vi "UHR-Fleezers Control (host) - 10.8.vi"() -> ()   [LabVIEW 2014] (continued)
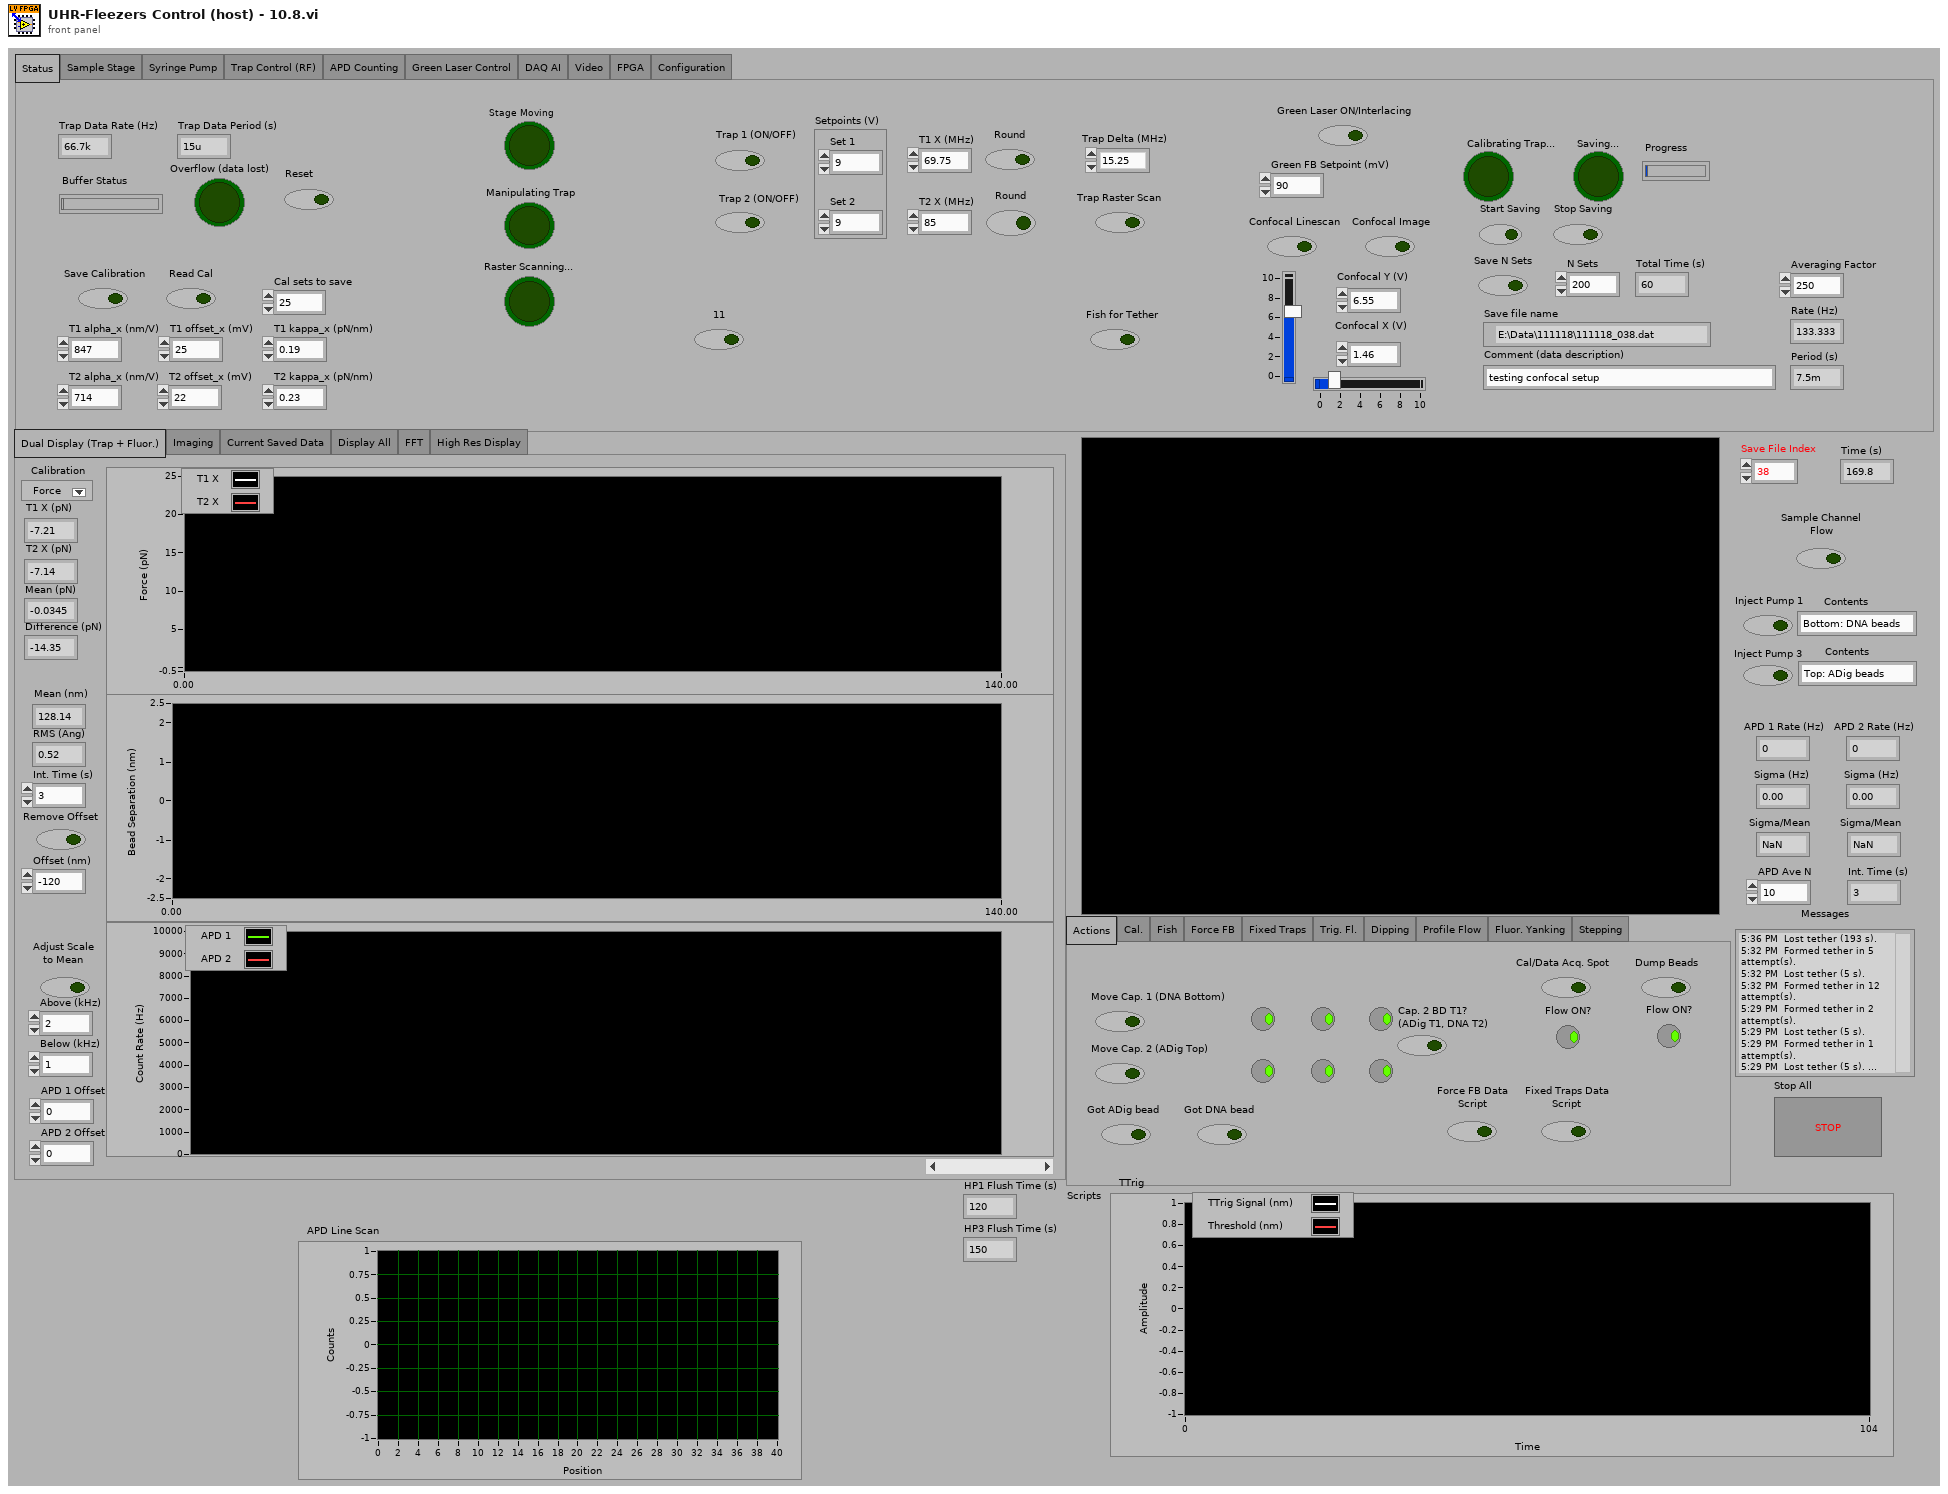
[diagram p1: front panel]
types:
  T1 = enum32{"Actions", "Cal.", "Fish", "Force FB", "Fixed Traps", "Trig. Fl.", "Dipping", "Profile Flow", "Fluor. Yanking", "Stepping"}
  T2 = typedef "IMAQ Image.ctl" = refnum<image>
  T3 = enum32{"Dual Display (Trap + Fluor.)", "Imaging", "Current Saved Data", "Display All", "FFT", "High Res Display"}
  T4 = enum32{"Status", "Sample Stage", "Syringe Pump", "Trap Control (RF)", "APD Counting", "Green Laser Control", "DAQ AI", "Video", "FPGA", "Configuration"}
  T5 = cluster{"Pump 1":cluster{"Diameter (mm)":dbl, "Units":dbl, "Volume":dbl, "Rate":dbl}, "Pump 2":cluster{"Diameter (mm)":dbl, "Units":dbl, "Volume":dbl, "Rate":dbl}, "Pump 3":cluster{"Diameter (mm)":dbl, "Units":dbl, "Volume":dbl, "Rate":dbl}}
  T6 = enum32{"IR Laser Interlacing (Direct RF Board Control Method)", "AOD Raster Scan", "Feedback on Trap Intensity", "Feedback on Trap Position"}
  T7 = typedef "LVPoint32TypeDef.ctl" = cluster{"Horizontal":i32, "Vertical":i32}
  T8 = cluster{"Scan Range AOD (nm) 2":dbl, "Step Size AOD (nm) 2":dbl, "Scan Speed AOD (nm/s) 2":dbl, "Number of scans (AOD) 2":u16, "Label":string}[]
  T9 = cluster{"Set 1":cluster{"proportional gain (Kc)":i16, "integral gain (Kc*Ts/Ti)":i16, "derivative gain (Kc*Td/Ts)":i16}, "Set 2":cluster{"proportional gain (Kc)":i16, "integral gain (Kc*Ts/Ti)":i16, "derivative gain (Kc*Td/Ts)":i16}}
  T10 = cluster{"Trap 1":fxp<+/-,16,1>, "Trap 2":fxp<+/-,16,1>}
  T11 = cluster{"proportional gain (Kc)":fxp<+/-,16,8>, "integral gain (Kc*Ts/Ti)":fxp<+/-,16,8>, "derivative gain (Kc*Td/Ts)":fxp<+/-,16,8>}
  T12 = cluster{"output high":fxp<+/-,16,1>, "output low":fxp<+/-,16,1>}
  T13 = cluster{"Set 1":fxp<+/-,16,1>, "Set 2":fxp<+/-,16,1>}
  T14 = cluster{"proportional gain (Kc)":i16, "integral gain (Kc*Ts/Ti)":i16, "derivative gain (Kc*Td/Ts)":i16}
  T15 = cluster{"Set 1":bool, "Set 2":bool, "Set 3":bool}
  T16 = typedef "LVMinMaxIncTypeDef.ctl" = cluster{"Minimum":dbl, "Maximum":dbl, "Increment":dbl}
  T17 = typedef "Image Type" = u32
  T18 = typedef "nirio_resource_hc.ctl" = tag
  T19 = typedef "openfpgaref.8.6.ctl" = refnum<k20>
  T20 = cluster{"New Image":T2, "New Image":T2, "New Image":T2, "New Image":T2}
  T21 = typedef "XDNodeRunTimeDep.lvlib/timing_clust.ctl" = cluster{"Expected End [f-1]":u64, "Actual End [f-1]":u64, "Finished Late? [f-1]":bool, "Expected End [i-1]":u64, "Actual End [i-1]":u64, "Finished Late? [i-1]":bool, "Expected Start [i]":u64, "Actual Start [i]":u64, "Expected Start [f]":u64, "Actual Start [f]":u64, "Source Name":string, "Structure Name":string, "Period":i64, "Deadline":i64, "Offset":i64, "Start":i64, "Priority":i32, "Timeout":i32, "Mode":T22, "Wakeup Reason":T23, "Error":errorcluster, "Source Type":string, "Secondary Source Type":string, "Global End Time":u64, "Global Start Time":u64, "Frame Duration":u64, "Iteration Duration":u64, "Assigned CPU":i32, "I/O Scan Engine Mode":u32}
  T22 = typedef "XDNodeRunTimeDep.lvlib/nitl_modes.ctl" = enum32{"No Change", "Process missed periods, maintain original phase", "Discard missed periods, maintain original phase", "Process missed periods, ignore original phase", "Discard missed periods, ignore original phase"}
  T23 = typedef "XDNodeRunTimeDep.lvlib/wakeup.ctl" = enum32{"Normal", "Aborted", "Asynchronous wakeup", "Timing source error", "Timed loop error", "Timeout"}
  T24 = enum16{"big-endian, network order", "native, host order", "little-endian"}
  T25 = enum16{"open", "replace", "create", "open or create", "replace or create", "replace or create with confirmation"}
  T26 = cluster{"Scan Range AOD (nm) 2":dbl, "Step Size AOD (nm) 2":dbl, "Scan Speed AOD (nm/s) 2":dbl, "Number of scans (AOD) 2":u16, "Label":string}
  T27 = cluster{"[0]":dbl, "[1]":dbl, "[2]":dbl, "[3]":dbl, "[4]":dbl, "[5]":dbl}
  T28 = cluster{"Diameter (mm)":dbl, "Units":dbl, "Volume":dbl, "Rate":dbl}
  T29 = cluster{"Left":i32, "Top":i32, "Width":u32, "Height":u32}
  T30 = cluster{cluster{"Left":i32, "Top":i32, "Width":u32, "Height":u32}}[]
  T31 = enum32{"setting", "request", "request control", "info", "statistics", "system settings", "I/O sub system", "HRT control", "camera descriptions", "device specific data", "event sub system settings", "event sub system results", "image memory manager"}
  T32 = typedef "AviRefnum.ctl" = refnum<k1>
  T33 = typedef "imagedata.ctl" = cluster{"image type":i32, "image depth":i32, "image":u8[], "mask":u8[], "colors":u32[], "Rectangle":cluster{"left":i16, "top":i16, "right":i16, "bottom":i16}}
  T34 = enum32{"Normal Display", "Dual Display (APD)", "FFT", "High Res Display"}
  T35 = cluster{"Origin Pixel":cluster{"X":sgl, "Y":sgl}, "Angle Relative to Horizontal (deg)":sgl, "Axis Reference":u32}
  T36 = typedef "Simple Grid Descriptor" = cluster{"X Step":sgl, "Y Step":sgl, "Unit":T37}
  T37 = typedef "Image Unit" = enum32{"Undefined", "Angström", "Micrometer", "Millimeter", "Centimeter", "Meter", "Kilometer", "Microinch", "Inch", "Feet", "Nautical miles", "Standard miles", "Steps"}
  T38 = cluster{"averaging mode":u16, "weighting mode":u16, "number of averages":u32}
  T39 = cluster{"dB On (F)":bool, "unwrap phase (F)":bool, "convert to degree (F)":bool}
  T40 = cluster{string, string, string, string, string, string, string, string}
  T41 = cluster{string, string, string, string, string, string, string, string, string, string, string, string}
  T42 = cluster{string, string, string, string, string, string, string, string, string, string, string, string, string}
  T43 = cluster{string, string, string, string, string, string, string, string, string, string, string, string, string, string}
  T44 = cluster{"BD 1 Frequency 1 (MHz)":dbl, "BD 1 Frequency 2 (MHz)":dbl}
  T45 = cluster{"f0":dbl, "df":dbl, "magnitude":dbl[]}[][]
diagram:
  w6 = u16 20 items=["1.0"=10, "1.5"=15, "2.0"=20] ("stop bits (10: 1 bit)")
  w9 = u16 20 items=["1.0"=10, "1.5"=15, "2.0"=20] ("stop bits (10: 1 bit)")
  w67 = u16 20 items=["1.0"=10, "1.5"=15, "2.0"=20] ("stop bits (10: 1 bit)")
  w74 = T17 2 items=["Grayscale (U8)", "Grayscale (I16)", "Grayscale (SGL)", "Complex (CSG)", "RGB (U32)", "HSL (U32)", "RGB (U64)", "Grayscale (U16)"] ("Image Type")
  w137 = cluster{"output high":i16, "output low":i16} {"output high"=3000, "output low"=0} ("FB output range 1")
  w208 = 10.0 ("y")
  w207 = 32767.0 ("y")
  w223 = 6.0  # clock mult.
  w224 = 49152000.0  # TCXO frequ.
  # "Bottom 1 Harvard"
  # "Top 3 Harvard"
  # "Center Harvard"
  # "Bottom 1 Harvard"
  # "Top 3 Harvard"
  # "Center Harvard"
  n1 = Build Array("DIO count 1 (ticks)", "DIO count 2 (ticks)", "DIO count 3 (ticks)") -> (w124:u32[])
  n2 = local read "AO1"() -> (w202:dbl)
  n3 = local read "AO2"() -> (w201:dbl)
  n4 = local read "Scan Increment (MHz)"() -> (w219:dbl)
  n5 = local read "Continuous MCL Scanning"() -> (w189:bool)
  n6 = local read "Fast Scan Dir"() -> (w188:bool)
  n7 = local read "Number of scans (MCL)"() -> (w190:u64)
  n8 = property on="AI Count (ticks)" class="DigNum (strict)"("Val(Sgnl)"="AI Count (ticks)") -> ()  [unwired: 2 in, 2 out]
  n9 = Multiply(x=w202, y=w207) -> (x*y=w204:dbl)
  n10 = Multiply(x=w201, y=w207) -> (x*y=w206:dbl)
  n11 = Divide(x=w204, y=w208) -> (x/y=w203:dbl)
  n12 = Divide(x=w206, y=w208) -> (x/y=w205:dbl)
  n13 = To Word Integer(number=w203) -> (16bit integer=w200:i16)
  n14 = To Word Integer(number=w205) -> (16bit integer=w199:i16)
  n15 = Not(x=w188) -> (.not. x?=w183:bool)
  n16 = local read "Cycles/step (MCL)"() -> (w191:u64)
  n17 = Multiply(x=w219, y=1000.0) -> (x*y=w226:dbl)
  n18 = local read "Scan steps (MCL)"() -> (w192:u64)
  n19 = local write "Trap Pos FIFO Timeout"(u16 0 ("Trap Pos FIFO Timeout")) -> ()
  n20 = local read "Desired Scan Incr (V)"() -> (w194:dbl)
  n21 = Scale By Power Of 2(n=48, x=w226) -> (x*2^n=w227:dbl)
  n22 = Multiply(x=w224, y=w223) -> (x*y=w222:dbl)
  n23 = Divide(x=w227, y=w222) -> (x/y=w221:dbl)
  n24 = local read "Setpoints (V)"() -> (w240:cluster{"Set 1":dbl, "Set 2":dbl})
  n25 = To Quad Integer(1:w221) -> (0:w218:i64)
  n26 = Divide(x=40000000.0, y="AI Count (ticks)") -> (x/y=w179:dbl)
  n27 = Multiply(x=w194, y=32767.0) -> (x*y=w196:dbl)
  n28 = local read "Number Interlace Sets"() -> (w117:u8)
  n29 = Split 1D Array(array=w124, index=w117) -> (first subarray=w126:u32[])  [unwired: 1 out]
  n30 = Add Array Elements(numeric array=w126) -> (sum=w125:u32)
  n31 = local read "# Samples/channel"() -> (w211:u32)
  n32 = local read "Number of F/B Scans (AOD)"() -> (w212:u16)
  n33 = local read "Not-Interlacing Set"() -> (w116:enum32{"Set 1", "Set 2", "Set 3"})
  n34 = To Unsigned Byte Integer(number=w116) -> (unsigned 8bit integer=w122:u8)
  n35 = Index Array(array=w124, index=w122) -> (element=w123:u32)
  n36 = local read "Feedback On/Off"() -> (w243:cluster{"Set 1":bool, "Set 2":bool})
  n37 = local read "PID Gains"() -> (w235:T9)
  n38 = local read "Scan steps (AOD)"() -> (w217:u64)
  n39 = local read "All FB On/Off"() -> (w244:bool)
  n40 = local read "Cycles/step (AOD)"() -> (w216:u64)
  n41 = local write "AI rate (Hz)"(w179) -> ()
  n42 = Divide(x=w196, y=10.0) -> (x/y=w195:dbl)
  n43 = Multiply(x=w217, y=w216) -> (x*y=w215:u64)
  n44 = Multiply(x=3276.7, y=w240) -> (x*y=w239:cluster{"Set 1":dbl, "Set 2":dbl})
  n45 = xnode "FPGA Open VI Reference"("resource name"=T18 "750kHzDAQ") -> ("FPGA VI Reference Out"=w232:T19, "error out"=w231:errorcluster)  [unwired: 1 in]
  n46 = To Word Integer(number=w195) -> (16bit integer=w193:i16)
  n47 = Multiply(x=w215, y=u64 2) -> (x*y=w213:u64)
  n48 = local read "Sets to FIFO (Traps)"() -> (w247:T15)
  n49 = Divide(x=w179, y="FPGA Ave.") -> (x/y=w180:dbl)
  n50 = To Word Integer(number=w239) -> (16bit integer=w238:cluster{"Set 1":i16, "Set 2":i16})
  n51 = Unbundle By Name(w235) -> ("Set 1"=w234:T14, "Set 2"=w233:T14)
  n52 = Multiply(x=w213, y=w212) -> (x*y=w210:u64)
  n53 = local write "Ave. Rate (Hz)"(w180) -> ()
  n54 = Divide(x=w210, y=w211) -> (x/y=w209:dbl)
  n55 = Unbundle By Name(w238) -> ("Set 1"=w237:i16, "Set 2"=w236:i16)
  n56 = local read "2D or 1D Scan"() -> (w138:bool)
  n57 = local write "Data points/scans"(w210) -> ()
  n58 = local read "Scan BD"() -> (w228:bool)
  n59 = And(x=w243, y=w244) -> (x .and. y?=w242:cluster{"Set 1":bool, "Set 2":bool})
  n60 = local write "Data points/scan (f/b)"(w213) -> ()
  n61 = Reciprocal(x=w180) -> (1/x=w181:dbl)
  n62 = local read "N Acq Sets (Traps + Fl.)"() -> (w172:i16)
  n63 = local write "N sets should be saved"(w209) -> ()
  n64 = xnode "Invoke Method"("FPGA VI Reference In"=w232, "error in"=w231) -> ("FPGA VI Reference Out"=w136:T19, "error out"=w146:errorcluster)
  n65 = Unbundle By Name(w242) -> ("Set 1"=w246:bool, "Set 2"=w245:bool)
  n66 = local read "Interlace"() -> (w118:bool)
  n67 = Select(t=w125, s=w118, f=w123) -> (s? t:f=w115:u32)
  n68 = local write "Update Count (MCL)"(w115) -> ()
  n69 = local write "Total Counts (ticks)"(w115) -> ()
  n70 = local write "Ave. Period (s)"(w181) -> ()
  n71 = property on="2D or 1D Scan" class="Bool (strict)"("Val(Sgnl)"=w138) -> ()  [unwired: 2 in, 2 out]
  n72 = local read "GI Frequency, OFF count"() -> (w38:u32)
  n73 = local read "GI Frequency, ON count"() -> (w29:u32)
  n74 = local read "APD Gate OFF Count"() -> (w35:u32)
  n75 = local read "APD Gate ON Count"() -> (w31:u32)
  n76 = xnode "Read/Write Control"("FPGA VI Reference In"=w135, "error in"=w146, "ai count"="AI Count (ticks)", "Interlace ON/OFF"=w118, "Number Interlace Cycles"=w117, "AI1 Sets to FIFO"=w247, "FB On/Off Set 1"=w246, "FB On/Off Set 2"=w245, "Interlace Off Parameters"=w116, "FB Setpoint Set 1"=w237, "FB Setpoint Set 2"=w236, "FB Gains Set 1"=w234, "FB Gains Set 2"=w233, "FB output range 1"=w137, "FB output range 2"=w137, "Cycles per step"=w216, "Scan BD"=w228, "Number of scans"=w212, "Scan steps"=w217, "Scan freq.  increment"=w218, "AO1"=w200, "AO2"=w199, "Scan freq.  increment (MCL)"=w193, "Scan steps (MCL)"=w192, "Cycles per step (MCL)"=w191, "Number of scans (MCL)"=w190, "MCL count"=w115, "Cont. Scan (MCL)"=w189, "MCL Scan Axis"=w183, "1D or 2D Scan?"=w138, "N of AI1 Int Acq Sets"=w172, "Freq or Amp switch first"="Freq or Amp switch first", "Freq switch delay"="Freq switch delay", "Amp switch delay"="Amp switch delay", "Swap F1 and F2"="Swap F1 and F2", "APD to FIFO"=FALSE, "DIO count 1 (ticks)"="DIO count 1 (ticks)", "DIO count 2 (ticks)"="DIO count 2 (ticks)", "DIO count 3 (ticks)"="DIO count 3 (ticks)") -> ("FPGA VI Reference Out"=w42:T19, "error out"=w40:errorcluster)  [unwired: 1 in]
  n77 = local read "On one out of X cycles"() -> (w37:u32)
  n78 = local read "APD Integration Time (s)"() -> (w21:dbl)
  n79 = local read "DMA Update Period (s)"() -> (w20:dbl)
  n80 = Add(x=w31, y=w35) -> (x+y=w33:u32)
  n81 = Add(x=w29, y=w38) -> (x+y=w36:u32)
  n82 = local read "Green Laser ON/Interlacing"() -> (w113:bool)
  n83 = local read "Green laser mode"() -> (w114:enum32{"Laser ON", "Laser OFF", "Interlace"})
  n84 = Multiply(x=w33, y=w37) -> (x*y=w34:u32)
  n85 = Multiply(x=w37, y=w36) -> (x*y=w28:u32)
  n86 = Reciprocal(x=w21) -> (1/x=w18:dbl)
  n87 = Multiply(x=w21, y=40000000.0) -> (x*y=w17:dbl)
  n88 = Divide(x=w20, y=w21) -> (x/y=w23:dbl)
  n89 = Multiply(x="Current When FB OFF (%)", y=655.35) -> (x*y=w101:dbl)
  n90 = local read "Invert APD Gate"() -> (w27:bool)
  n91 = Multiply(x="Green FB Setpoint (mV)", y=3.2767) -> (x*y=w98:dbl)
  n92 = local read "APD Gate"() -> (w26:enum32{"ON", "OFF", "Interlace"})
  n93 = Subtract(x=w34, y=w31) -> (x-y=w32:u32)
  n94 = local write "Green FB Count"(w28) -> ()
  n95 = local write "APD Acq Rate (Hz)"(w18) -> ()
  n96 = To Unsigned Long Integer(number=w17) -> (unsigned 32bit integer=w15:u32)
  n97 = Multiply(x=2.0, y=w23) -> (x*y=w22:dbl)
  n98 = local read "Invert GI"() -> (w110:bool)
  n99 = To Unsigned Word Integer(number=w101) -> (unsigned 16bit integer=w99:u16)
  n100 = Subtract(x=w28, y=w29) -> (x-y=w30:u32)
  n101 = local write "APD Samples/FIFO Acq."(w23) -> ()
  n102 = To Word Integer(number=w98) -> (16bit integer=w96:i16)
  n103 = local write "APD Elements/DMA read"(w22) -> ()
  n104 = case shown="False" w113 {
    tunnel: w114 -> [_ w273]
    tunnel: [enum32{"Laser ON", "Laser OFF", "Interlace"}."Laser OFF" ("Green laser mode") w273] -> w109
    frame False {
    }
    frame True {
    }
  }
  n105 = local write "APD Int. Count"(w15) -> ()
  n106 = local read "Trap Pos. AI1 X Pre-scale"() -> (w53:u16)
  n107 = local read "Trap Pos FB Monitor\nT1 or T2"() -> (w60:bool)
  n108 = local read "Trap Pos FB Int Count"() -> (w46:u16)
  n109 = local read "APD 1 AO Mult."() -> (w25:i16)
  n110 = local read "Trap Pos FB Negate Action"() -> (w59:bool)
  n111 = local read "APD 2 AO Mult."() -> (w24:i16)
  n112 = local read "Trap Pos. FB Offset Factor"() -> (w58:i64)
  n113 = local read "Trap Pos. FB Mult Factor"() -> (w57:i64)
  n114 = local read "Differential FB?"() -> (w12:bool)
  n115 = local read "Neg. TTrig FPGA"() -> (w14:bool)
  n116 = local read "Trap Pos. FB Gains"() -> (w55:T11)
  n117 = local read "Trap Pos. FB Range"() -> (w56:T12)
  n118 = xnode "Read/Write Control"("FPGA VI Reference In"=w42, "error in"=w40, "Invert APD Gate"=w27, "APD Gate ON Count"=w31, "APD Gate OFF Count"=w32, "APD Acq Rate Count"=w15, "APD Gate Operating Mode"=w26, "APD 1 AO scale factor"=w25, "APD 2 AO scale factor"=w24, "Green interlace ON count"=w29, "Green interlace OFF count"=w30, "Green interlace ON count 2"=w29, "Green interlace OFF count 2"=w30, "Green FB Count"=w28) -> ("FPGA VI Reference Out"=w41:T19, "error out"=w39:errorcluster)
  n119 = xnode "Read/Write Control"("FPGA VI Reference In"=w41, "error in"=w39, "Invert GI 2"=w110, "Operating Mode 2"=w109, "Green FB Gains"="Green FB Gains", "Green FB Setpoint"=w96, "Green FB On/Off"="Green FB On/Off", "Current Out"=w99, "Green int current ON count adj"="Green int current ON count adj", "Operating Mode"=w109, "Invert GI"=w110, "Trap Pos FB Monitor T1 or T2"=w60, "Trap Pos FB Negate Action"=w59, "Trap Pos. FB Offset Factor"=w58, "Trap Pos. FB Mult Factor"=w57, "Trap Pos. FB Range"=w56, "Trap Pos. FB Gains"=w55, "Force feedback"=FALSE, "AI1 X Scale"=w53, "Trap Pos to FIFO"=TRUE, "Trap Pos FB Int Count"=w46, "TTrig Negate Pos"=w14, "FB Trig Integrate"="FB Trig Integrate", "Diff FB Measurement?"=w12, "Negate Diff?"="Negate Diff?") -> ("FPGA VI Reference Out"=w111:T19, "error out"=w112:errorcluster)
  n120 = xnode "Invoke Method"("FPGA VI Reference In"=w111, "error in"=w112, "Requested Depth"="Trap AI FIFO Depth") -> ("FPGA VI Reference Out"=w63:T19, "error out"=w62:errorcluster)  [unwired: 1 out]
  n121 = xnode "Invoke Method"("FPGA VI Reference In"=w63, "error in"=w62, "Requested Depth"="Trap Position FIFO Depth") -> ("FPGA VI Reference Out"=w48:T19, "error out"=w47:errorcluster)  [unwired: 1 out]
  n122 = flat-sequence {
    tunnel: w136 -> [w278]
    tunnel: [w278] -> w135
    tunnel: [w277] -> w134
    tunnel: [w276] -> w133
    tunnel: [w274] -> w131
    tunnel: [w275] -> w132
    frame #0 {
      w275 = T16 {"Minimum"=0.0, "Maximum"=40.0, "Increment"=1.0} ("Min Max Inc")
      w274 = T16 {"Minimum"=0.0, "Maximum"=50.0, "Increment"=1.0} ("Data Entry Limits")
      w277 = T16 {"Minimum"=60.0, "Maximum"=90.0, "Increment"=1.0} ("Min Max Inc")
      w276 = T16 {"Minimum"=0.0, "Maximum"=50.0, "Increment"=1.0} ("Data Entry Limits")
      n123 = property on="BD 2 Frequency 1 (MHz)" class="DigNum (strict)"("Data Range"=w275) -> ()  [unwired: 2 in, 2 out]
      n124 = property on="BD 2 Frequency 3 (MHz)" class="DigNum (strict)"("Data Range"=w275) -> ()  [unwired: 2 in, 2 out]
      n125 = property on="BD 2 Frequency 2 (MHz)" class="DigNum (strict)"("Data Range"=w275) -> ()  [unwired: 2 in, 2 out]
      n126 = property on="BD 1 Frequency 1 (MHz)" class="DigNum (strict)"("Data Range"=w277) -> ()  [unwired: 2 in, 2 out]
      n127 = property on="BD 1 Frequency 2 (MHz)" class="DigNum (strict)"("Data Range"=w277) -> ()  [unwired: 2 in, 2 out]
      n128 = property on="BD 1 Frequency 3 (MHz)" class="DigNum (strict)"("Data Range"=w277) -> ()  [unwired: 2 in, 2 out]
      n129 = property on="BD 2 Amplitude 1 (%)" class="DigNum (strict)"("Data Range"=w274) -> ()  [unwired: 2 in, 2 out]
      n130 = property on="BD 2 Amplitude 2 (%)" class="DigNum (strict)"("Data Range"=w274) -> ()  [unwired: 2 in, 2 out]
      n131 = property on="BD 2 Amplitude 3 (%)" class="DigNum (strict)"("Data Range"=w274) -> ()  [unwired: 2 in, 2 out]
      n132 = property on="BD 1 Amplitude 3 (%)" class="DigNum (strict)"("Data Range"=w276) -> ()  [unwired: 2 in, 2 out]
      n133 = property on="BD 1 Amplitude 2 (%)" class="DigNum (strict)"("Data Range"=w276) -> ()  [unwired: 2 in, 2 out]
      n134 = property on="BD 1 Amplitude 1 (%)" class="DigNum (strict)"("Data Range"=w276) -> ()  [unwired: 2 in, 2 out]
      "X RF Frequency Limits (MHz)" <- w277
      "X RF Amplitude Limits (%)" <- w276
      "Y RF Amplitude Limits (%)" <- w274
      "Y RF Frequency Limits (MHz)" <- w275
    }
  }
  n135 = xnode "Invoke Method"("FPGA VI Reference In"=w48, "error in"=w47) -> ("FPGA VI Reference Out"=w145:T19, "error out"=w144:errorcluster)  [unwired: 1 in]
  n136 = flat-sequence "Initial FPGA Loop Relative Phase Adjustment" {
    tunnel: "Initial Phase Adjustment (AI1)" -> [w289]
    tunnel: "Initial Phase Adjustment (GI)" -> [w288]
    tunnel: w145 -> [w287]
    tunnel: w144 -> [w286]
    tunnel: "Initial Phase Adj. (MCL)" -> [w285]
    tunnel: [w290] -> w154
    tunnel: [w284] -> w150
    tunnel: "Initial Phase Adjustment (APD Acq)" -> [w283]
    tunnel: "Initial Phase Adjustment (APD 1 Gate)" -> [w282]
    tunnel: "Initial Phase Adjustment (Green FB)" -> [w281]
    tunnel: "Initial Phase Adjustment (GI) 2" -> [w280]
    tunnel: "Initial Phase Adjustment (APD 2 Gate)" -> [w279]
    tunnel: w154 -> [w292]
    tunnel: [w293] -> w151
    tunnel: w150 -> [w293]
    tunnel: [w292] -> w149
    tunnel: w151 -> [w296]
    tunnel: w149 -> [w295]
    tunnel: [w298] -> w148
    tunnel: [w297] -> w147
    tunnel: [w300] -> w152
    tunnel: [w301] -> w153
    tunnel: w148 -> [w301]
    tunnel: w147 -> [w300]
    frame #0 {
      n137 = xnode "Read/Write Control"("FPGA VI Reference In"=w287, "error in"=w286, "Phase count adjustment"=w289, "Phase count adjustment (GI)"=w288, "Phase count adjustment (MCL)"=w285, "Phase Count Adjustment (APD Acq)"=w283, "Phase count adjustment (APD 1 Gate)"=w282, "Phase count adjustment (APD 2 Gate)"=w279, "Phase count adjustment (Green FB)"=w281, "Phase count adjustment (GI) 2"=w280) -> ("FPGA VI Reference Out"=w284:T19, "error out"=w290:errorcluster)
    }
    frame #1 {
      n138 = Wait (ms)(milliseconds to wait=u32 100) -> ()  [unwired: 1 out]
    }
    frame #2 {
      w294 = TRUE
      n139 = xnode "Read/Write Control"("FPGA VI Reference In"=w296, "error in"=w295, "+ phase"=w294, "+ phase (GI)"=w294, "+ phase (MCL)"=w294, "+ phase (APD Acq)"=w294, "+ phase (APD 1 Gate)"=w294, "+ phase (APD 2 Gate)"=w294, "+ phase (Green FB)"=w294, "+ phase (GI) 2"=w294) -> ("FPGA VI Reference Out"=w297:T19, "error out"=w298:errorcluster)
    }
    frame #3 {
      n140 = Wait (ms)(milliseconds to wait=u32 100) -> ()  [unwired: 1 out]
    }
  }
  n141 = local read "Phase adj. (Green FB)"() -> (w127:i16)
  n142 = local read "Phase adj. (GI) 2"() -> (w102:i16)
  n143 = local read "Phase adjust (MCL)"() -> (w184:i16)
  n144 = local read "Phase adj. (AI1)"() -> (w186:i16)
  n145 = local read "Phase adj. (GI)"() -> (w185:i16)
  n146 = xnode "Read/Write Control"("FPGA VI Reference In"=w152, "error in"=w153, "Phase count adjustment"=w186, "Phase count adjustment (GI)"=w185, "Phase count adjustment (MCL)"=w184, "Phase Count Adjustment (APD Acq)"="Phase Adj. (APD Acq)", "Phase count adjustment (APD 1 Gate)"="Phase Adj. (APD 1 Gate)", "Phase count adjustment (APD 2 Gate)"="Phase Adj. (APD 2 Gate)", "Phase count adjustment (Green FB)"=w127, "Phase count adjustment (GI) 2"=w102) -> ("FPGA VI Reference Out"=w88:T19, "error out"=w161:errorcluster)
  n147 = call "Initialize RF boards - interlace 3.vi"("error in"=w161, "FPGA VI Reference In"=w88) -> ("error out"=w159:errorcluster, "FPGA VI Reference Out"=w160:T19)
  n148 = call "set RF board frequency - interlace.vi"("Board 2 Frequency Limits"=w132, "Board 1 Frequency Limits"=w134, "error in"=w159, "FPGA VI Reference In"=w160, "Board 2 Frequency 3 (MHz)"="BD 2 Frequency 3 (MHz)", "Board 1 Frequency 3 (MHz)"="BD 1 Frequency 3 (MHz)", "Board 2 Frequency 2 (MHz)"="BD 2 Frequency 2 (MHz)", "Board 2 Frequency 1 (MHz)"="BD 2 Frequency 1 (MHz)", "Board 1 Frequency 2 (MHz)"="BD 1 Frequency 2 (MHz)", "Board 1 Frequency 1  (MHz)"="BD 1 Frequency 1 (MHz)") -> ("error out"=w262:errorcluster, "FPGA VI Reference Out"=w263:T19)
  n149 = call "set RF board amplitude - interlace.vi"("Board 2 Amplitude Limits"=w131, "Board 1 Amplitude Limits"=w133, "error in"=w262, "FPGA VI Reference In"=w263, "Board 2 Amplitude 3 (%)"="BD 2 Amplitude 3 (%)", "Board 1 Amplitude 3 (%)"="BD 1 Amplitude 3 (%)", "Board 2 Amplitude 2 (%)"="BD 2 Amplitude 2 (%)", "Board 2 Amplitude 1 (%)"="BD 2 Amplitude 1 (%)", "Board 1 Amplitude 2 (%)"="BD 1 Amplitude 2 (%)", "Board 1 Amplitude 1 (%)"="BD 1 Amplitude 1 (%)") -> ("error out"=w250:errorcluster, "FPGA VI Reference Out"=w251:T19)
  n150 = flat-sequence {
    tunnel: w251 -> [w311]
    tunnel: w250 -> [w310]
    tunnel: [w309] -> w255
    tunnel: [w308] -> w254
    tunnel: [w315] -> w253
    tunnel: w255 -> [w315]
    tunnel: [w314] -> w252
    tunnel: w254 -> [w314]
    tunnel: w253 -> [w324]
    tunnel: w252 -> [w323]
    tunnel: [w322] -> w50
    tunnel: [w321] -> w49
    frame #0 {
      w302 = FALSE ("Retract Pump 3")
      n151 = local read "Trap 1 (ON/OFF)"() -> (w303:bool)
      n152 = xnode "Read/Write Control"("FPGA VI Reference In"=w311, "error in"=w310, "Direct RF Box  Communication"=FALSE) -> ("FPGA VI Reference Out"=w309:T19, "error out"=w308:errorcluster)
      n153 = local write "Saving..."(FALSE ("Saving Data")) -> ()
      n154 = local write "Stop All"(FALSE ("Stop All")) -> ()
      n155 = local write "Retract Pump 1"(w302) -> ()
      n156 = local write "Retract Pump 3"(w302) -> ()
      n157 = local write "Index"(1.0 ("Index")) -> ()
      n158 = property on="Trap 1 ON" class="Bool (strict)"("Value"=w303) -> ()  [unwired: 2 in, 2 out]
      "Manipulating Trap" <- FALSE ("Manipulating Trap")
    }
    frame #1 {
      n159 = local read "Trap 2 (ON/OFF)"() -> (w313:bool)
      n160 = Wait (ms)(milliseconds to wait=u32 10) -> ()  [unwired: 1 out]
      n161 = property on="Trap 2 ON" class="Bool (strict)"("Val(Sgnl)"=w313) -> ()  [unwired: 2 in, 2 out]
    }
    frame #2 {
      n162 = local read "Scan Range (nm)"() -> (w317:dbl)
      n163 = xnode "Read/Write Control"("FPGA VI Reference In"=w324, "error in"=w323, "FPGA Controls  RF Box"=TRUE ("Direct RF Box  Communication")) -> ("FPGA VI Reference Out"=w322:T19, "error out"=w321:errorcluster)
      n164 = call "Update messages.vi"("Message to add"="UHR-Fleezers ready.", "Old message string"="") -> ("New message string"=w320:string)
      n165 = local write "Messages"(w320) -> ()
      n166 = property on="Scan Range (nm)" class="DigNum (strict)"("Val(Sgnl)"=w317) -> ()  [unwired: 2 in, 2 out]
    }
  }
  n167 = Subtract(x="BD 1 Frequency 1 (MHz)", y="BD 1 Frequency 2 (MHz)") -> (x-y=w171:dbl)
  n168 = Subtract(x="BD 2 Frequency 1 (MHz)", y="BD 2 Frequency 2 (MHz)") -> (x-y=w170:dbl)
  n169 = Square(x=w170) -> (x^2=w168:dbl)
  n170 = Square(x=w171) -> (x^2=w169:dbl)
  n171 = Add(x=w169, y=w168) -> (x+y=w167:dbl)
  n172 = Square Root(x=w167) -> (sqrt(x)=w166:dbl)
  n173 = local write "Trap Delta (MHz)"(w166) -> ()
  n174 = call "IMAQ Create"("Image Name"="APD 1 Image", "Image Type"=w74) -> ("New Image"=w73:T2)  [unwired: 3 in, 1 out]
  n175 = call "IMAQ Create"("Image Name"="APD 2 Image", "Image Type"=w74) -> ("New Image"=w72:T2)  [unwired: 3 in, 1 out]
  n176 = call "IMAQ Create"("Image Name"="Det. X Image", "Image Type"=w74) -> ("New Image"=w71:T2)  [unwired: 3 in, 1 out]
  n177 = call "IMAQ Create"("Image Name"="Det. Y Image", "Image Type"=w74) -> ("New Image"=w70:T2)  [unwired: 3 in, 1 out]
  n178 = Bundle("New Image"=w73, "New Image"=w72, "New Image"=w71, "New Image"=w70) -> (w69:T20)  [unwired: 1 in]
  n179 = call-poly "VISA Configure Serial Port"("VISA resource name"="Bottom  1 Harvard Syringe Pump Serial Port", "baud rate (9600)"=u32 115200, "stop bits (10: 1 bit)"=w6) -> ("VISA resource name out"=w2:refnum<visa-resource-name>, "error out"=w1:errorcluster)  [unwired: 4 in, 7 out]
  n180 = call-poly "VISA Configure Serial Port"("VISA resource name"="Top 3 Harvard Syringe Pump Serial Port", "baud rate (9600)"=u32 115200, "stop bits (10: 1 bit)"=w9) -> ("VISA resource name out"=w4:refnum<visa-resource-name>, "error out"=w3:errorcluster)  [unwired: 4 in, 7 out]
  n181 = call-poly "VISA Configure Serial Port"("VISA resource name"="Sample Chamber Stage Serial Port") -> ("VISA resource name out"=w83:refnum<visa-resource-name>, "error out"=w84:errorcluster)  [unwired: 5 in, 8 out]
  "Stage Control Serial Error" <- w84
  n182 = call-poly "VISA Configure Serial Port"("VISA resource name"="Center Harvard Syringe Pump Serial Port", "baud rate (9600)"=u32 115200, "stop bits (10: 1 bit)"=w67) -> ("VISA resource name out"=w64:refnum<visa-resource-name>, "error out"=w65:errorcluster)  [unwired: 4 in, 7 out]
  n183 = disable-structure shown="Disabled" {
    disable-tunnel: [w327 _] -> w230
    disable-tunnel: w50 -> [w326 _]
    frame Disabled {
      n184 = node-c288() -> (w329:T21)  [unwired: 4 out]
      n185 = timed-loop "Rough control of MCL mirror stage (debugging)" {
        tunnel: w326 -> [w332]
        tunnel: [w331] -> w327
        timing: w329 -> [_]
        timing-out: [_] -> w328
        stop <- w331 stop-if-true
        n186 = node-c288() -> ()  [unwired: 2 out]
        n187 = case shown="1" "MCL Mode" {
          tunnel: w332 -> [_ w335 w382]
          frame 0, Default {
          }
          frame 1 {
            n188 = node-c288() -> (w337:T21)  [unwired: 4 out]
            n189 = timed-loop "Oscillate MCL mirror" {
              timing: w337 -> [_]
              timing-out: [_] -> w336
              tunnel: w335 -> [w376]
              i -> [w375]
              stop <- w338 stop-if-true
              n190 = node-c288() -> (w374:i64)  [unwired: 1 out]
              n191 = Multiply(x="AO1", y=32767.0) -> (x*y=w370:dbl)
              n192 = Multiply(x="AO2", y=32767.0) -> (x*y=w365:dbl)
              n193 = Divide(x=w370, y=10.0) -> (x/y=w371:dbl)
              n194 = Divide(x=w365, y=10.0) -> (x/y=w366:dbl)
              n195 = To Word Integer(number=w371) -> (16bit integer=w363:i16)
              n196 = To Word Integer(number=w366) -> (16bit integer=w362:i16)
              n197 = Divide(x=w374, y=i64 1000) -> (x/y=w345:dbl)
              n198 = Multiply(x=w345, y=w375) -> (x*y=w356:dbl)
              n199 = Multiply(x="Osc. freq. (Hz) 2", y=6.283185307179586) -> (x*y=w357:dbl)
              n200 = Multiply(x=w357, y=w356) -> (x*y=w355:dbl)
              n201 = Sine(x=w355) -> (sin(x)=w354:dbl)
              n202 = Multiply(x=w354, y="Osc. amp. (V)") -> (x*y=w352:dbl)
              n203 = Add(x=w352, y="Osc. center (V)") -> (x+y=w350:dbl)
              n204 = Divide(x=w350, y=10.0) -> (x/y=w348:dbl)
              n205 = Multiply(x=w348, y=32767.0) -> (x*y=w343:dbl)
              n206 = Select(t=w343, s="Scan axis", f=w363) -> (s? t:f=w361:dbl)
              n207 = Select(t=w362, s="Scan axis", f=w343) -> (s? t:f=w360:dbl)
              n208 = local read "MCL Mode"() -> (w342:u16)
              n209 = Not Equal?(x=w342, y=u16 1) -> (x != y?=w339:bool)
              n210 = local read "Stop All"() -> (w340:bool)
              n211 = xnode "Read/Write Control"("FPGA VI Reference In"=w376, "AO1"=w361, "AO2"=w360) -> ()  [unwired: 1 in, 2 out]
              n212 = Compound Arithmetic op=OR(w340, w339) -> (w338:bool)
              n213 = node-c288() -> ()  [unwired: 2 out]
            }
            n214 = node-c288(w336) -> ()  [unwired: 1 out]
          }
          frame 2 {
            n215 = case shown="True" "Start Scan" {
              tunnel: w382 -> [_ w394]
              frame False {
              }
              frame True {
                n216 = Subtract(x="End (V)", y="Begin (V)") -> (x-y=w390:dbl)
                n217 = Decrement(x="N Points") -> (x-1=w389:dbl)
                n218 = Divide(x=w390, y=w389) -> (x/y=w387:dbl)
                n219 = for {
                  N: "N Points" -> [_]
                  tunnel: "Begin (V)" -> [w407]
                  tunnel: w394 -> [w399]
                  tunnel: [w398] -> w393 mode=indexing
                  tunnel: w387 -> [w397]
                  tunnel: [w395] -> w386 mode=indexing
                  i -> [w406]
                  n220 = Multiply(x=w397, y=w406) -> (x*y=w405:dbl)
                  n221 = Add(x=w407, y=w405) -> (x+y=w402:dbl)
                  n222 = local read "Scan axis"() -> (w396:bool)
                  n223 = local read "AO1"() -> (w404:dbl)
                  n224 = local read "AO2"() -> (w403:dbl)
                  n225 = Select(t=w402, s=w396, f=w404) -> (s? t:f=w401:dbl)
                  n226 = Select(t=w403, s=w396, f=w402) -> (s? t:f=w400:dbl)
                  n227 = flat-sequence {
                    tunnel: w401 -> [w411]
                    tunnel: w400 -> [w410]
                    tunnel: w399 -> [w408]
                    tunnel: [w421] -> w398
                    tunnel: [w420] -> w395
                    frame #0 {
                      w414 = 10.0 ("y")
                      w409 = 32767.0 ("y")
                      n228 = Multiply(x=w411, y=w409) -> (x*y=w417:dbl)
                      n229 = Multiply(x=w410, y=w409) -> (x*y=w415:dbl)
                      n230 = Divide(x=w417, y=w414) -> (x/y=w418:dbl)
                      n231 = Divide(x=w415, y=w414) -> (x/y=w416:dbl)
                      n232 = To Word Integer(number=w418) -> (16bit integer=w412:i16)
                      n233 = To Word Integer(number=w416) -> (16bit integer=w413:i16)
                      n234 = xnode "Read/Write Control"("FPGA VI Reference In"=w408, "AO1"=w412, "AO2"=w413) -> ()  [unwired: 1 in, 2 out]
                    }
                    frame #1 {
                      n235 = Wait (ms)(milliseconds to wait="DAQ Delay (ms)") -> ()  [unwired: 1 out]
                    }
                    frame #2 {
                      n236 = local read "Slow mean"() -> (w421:dbl)
                      n237 = local read "Sigma"() -> (w420:dbl)
                    }
                  }
                }
                n238 = Bundle("Begin (V)"="Begin (V)", w387, w393) -> (→"MCL Scan":cluster{"Begin (V)":dbl, dbl, dbl[]})  [unwired: 1 out]
                n239 = Bundle("Begin (V)"="Begin (V)", w387, w386) -> (→"MCL Scan 2":cluster{"Begin (V)":dbl, dbl, dbl[]})  [unwired: 1 out]
              }
            }
          }
        }
        n240 = local read "Stop All"() -> (w331:bool)
        n241 = node-c288() -> ()  [unwired: 2 out]
      }
      n242 = node-c288(w328) -> ()  [unwired: 1 out]
    }
    frame Enabled {
    }
  }
  n243 = node-c288(3 ("Processor")) -> (w90:T21)  [unwired: 3 out]
  n244 = timed-loop "Oscillate Trap/AOM (fishing, debugging)" {
    tunnel: w50 -> [w425]
    tunnel: [w424] -> w95
    timing: w90 -> [_]
    timing-out: [_] -> w89
    stop <- w424 stop-if-true
    n245 = node-c288() -> ()  [unwired: 2 out]
    n246 = event shown="[1] \"Fl. Triggered...\": Value Change" {
      selector: _ -> [_ _ _]
      dyn-events: _ -> [_ _ _]
      timeout: _ -> [_ _ _]
      tunnel: w425 -> [w432 _ _]
      tunnel: [FALSE ("Stop All") _ w920] -> w424
      event "Oscillate Set 1", "Fish for Tether": Value Change {
        n247 = event-data() -> ()  [unwired: 6 out]
        n248 = local read "Oscillate Set 1"() -> (w431:bool)
        n249 = Or(x=w431, y="Fish for Tether") -> (x .or. y?=w429:bool)
        n250 = case shown="True" w429 {
          tunnel: w432 -> [_ w435]
          tunnel: "Fish for Tether" -> [_ w434]
          frame False {
          }
          frame True {
            n251 = case shown="True" w434 {
              selector: w434 -> [w438 w444]
              tunnel: [w438 w444] -> w433
              frame False {
              }
              frame True {
                n252 = local write "Scan axis 2"(TRUE) -> ()
                n253 = local write "Tether"(FALSE ("Tether")) -> ()
                n254 = local read "Flow ON during cal?"() -> (w439:bool)
                n255 = property on="Trap Delta (MHz)" class="DigNum (strict)"("Val(Sgnl)"="Furthest Delta (MHz)") -> ()  [unwired: 2 in, 2 out]
                n256 = Or(x="Flow ON during \nfishing?", y=w439) -> (x .or. y?=w440:bool)
                n257 = Wait (ms)(milliseconds to wait=u32 500) -> ()  [unwired: 1 out]
                n258 = property on="Sample Channel\nFlow" class="Bool (strict)"("Val(Sgnl)"=w440) -> ()  [unwired: 2 in, 2 out]
              }
            }
            n259 = node-c288() -> (w437:T21)  [unwired: 4 out]
            n260 = timed-loop "Oscillate AOD" {
              timing: w437 -> [_]
              timing-out: [_] -> w436
              tunnel: w435 -> [w454]
              tunnel: w433 -> [w447]
              i -> [w456]
              stop <- w453 stop-if-true
              n261 = node-c288() -> (w455:i64)  [unwired: 1 out]
              n262 = flat-sequence {
                tunnel: w456 -> [w483]
                tunnel: w455 -> [w482]
                tunnel: w454 -> [w461]
                tunnel: w447 -> [w464]
                tunnel: [w464] -> w452
                tunnel: [w463] -> w451
                tunnel: [w460] -> w450
                tunnel: [w457] -> w448
                tunnel: w452 -> [w519]
                tunnel: w451 -> [w517]
                tunnel: w450 -> [w516]
                tunnel: [w515] -> w449
                tunnel: w448 -> [w514]
                tunnel: [w591] -> w453
                tunnel: w449 -> [w590]
                frame #0 {
                  n263 = Divide(x=w482, y=i64 1000) -> (x/y=w477:dbl)
                  n264 = Multiply(x=w477, y=w483) -> (x*y=w479:dbl)
                  n265 = local read "BD 1 Frequency 2 (MHz)"() -> (w462:dbl)
                  n266 = Multiply(x="Osc. freq. (Hz)", y=6.283185307179586) -> (x*y=w480:dbl)
                  n267 = Multiply(x=w480, y=w479) -> (x*y=w459:dbl)
                  n268 = local read "BD 1 Frequency 1 (MHz)"() -> (w467:dbl)
                  n269 = local read "BD 2 Frequency 1 (MHz)"() -> (w466:dbl)
                  n270 = case shown="True" w464 {
                    tunnel: w459 -> [w489 w494]
                    tunnel: w467 -> [_ w505]
                    tunnel: w462 -> [_ w506]
                    tunnel: [w486 w500] -> w465
                    tunnel: [FALSE w497] -> w460
                    tunnel: [0.0 w490] -> w457
                    frame False {
                      n271 = Sine(x=w489) -> (sin(x)=w487:dbl)
                      n272 = Multiply(x=w487, y="Osc. amp. (MHz)") -> (x*y=w486:dbl)
                    }
                    frame True {
                      n273 = Cosine(x=w494) -> (cos(x)=w509:dbl)
                      n274 = Subtract(x=w506, y=w505) -> (x-y=w504:dbl)
                      n275 = Decrement(x=w509) -> (x-1=w508:dbl)
                      n276 = Subtract(x=w504, y="Closest Delta (MHz)") -> (x-y=w501:dbl)
                      n277 = Divide(x=w508, y=-2.0) -> (x/y=w502:dbl)
                      n278 = Multiply(x=w502, y=w501) -> (x*y=w500:dbl)
                      n279 = local read "Vec Mean of T1 T2"() -> (w496:dbl[])
                      n280 = Greater?(x=w496, y="Stop F (pN)") -> (0:w498:bool[])
                      n281 = Or Array Elements(Boolean array=w498) -> (logical OR=w497:bool)
                      n282 = Divide(x=w494, y=6.283185307179586) -> (x/y=w493:dbl)
                      n283 = Round Toward +Infinity(x=w493) -> (ceil(x): smallest int >= x=w490:dbl)
                      "Attempts" <- w490
                      n284 = Greater?(x=w490, y="Attempt Limit") -> (0:w492:bool)
                      n285 = case shown="True" w492 {
                        frame False {
                        }
                        frame True {
                          n286 = local write "Fish for Tether"(FALSE ("Fish for Tether")) -> ()
                          n287 = call <vilib>:"Beep.vi"() -> ()  [unwired: 3 in, 9 out]
                          n288 = local read "Messages"() -> (w511:string)
                          n289 = call "Update messages.vi"("Message to add"="Tether fishing timeout." ("Messages"), "Old message string"=w511) -> ("New message string"=→"Messages":string)
                        }
                      }
                    }
                  }
                  n290 = Select(t=w467, s="Scan axis 2", f=w466) -> (s? t:f=w470:dbl)
                  n291 = Add(x=w465, y=w470) -> (x+y=w463:dbl)
                  n292 = Select(t=w463, s="Scan axis 2", f=w467) -> (s? t:f=w473:dbl)
                  n293 = Select(t=w466, s="Scan axis 2", f=w463) -> (s? t:f=w472:dbl)
                  n294 = local read "Y RF Frequency Limits (MHz)"() -> (w468:T16)
                  n295 = local read "X RF Frequency Limits (MHz)"() -> (w469:T16)
                  n296 = local read "BD 1 Frequency 3 (MHz)"() -> (w476:dbl)
                  n297 = local read "BD 2 Frequency 2 (MHz)"() -> (w475:dbl)
                  n298 = local read "BD 2 Frequency 3 (MHz)"() -> (w474:dbl)
                  n299 = call "set RF board frequency - interlace.vi"("Board 2 Frequency Limits"=w468, "Board 1 Frequency Limits"=w469, "FPGA VI Reference In"=w461, "Board 2 Frequency 3 (MHz)"=w474, "Board 1 Frequency 3 (MHz)"=w476, "Board 2 Frequency 2 (MHz)"=w475, "Board 2 Frequency 1 (MHz)"=w472, "Board 1 Frequency 2 (MHz)"=w462, "Board 1 Frequency 1  (MHz)"=w473) -> ()  [unwired: 1 in, 2 out]
                }
                frame #1 {
                  n300 = And(x=w519, y=w516) -> (x .and. y?=w518:bool)
                  n301 = case "Only if were fishing and now formed tether" shown="True" w518 {
                    tunnel: w517 -> [w521 w536]
                    tunnel: [w520 w535] -> w515
                    tunnel: w514 -> [_ w531]
                    frame False {
                      n302 = local read "Fish for Tether"() -> (w520:bool)
                      n303 = case shown="False" w520 {
                        tunnel: w521 -> [w522 _]
                        frame False {
                          n304 = property on="BD 1 Frequency 1 (MHz)" class="DigNum (strict)"("Val(Sgnl)"=w522) -> ()  [unwired: 2 in, 2 out]
                        }
                        frame True {
                        }
                      }
                    }
                    frame True {
                      w535 = FALSE ("Fish for Tether")
                      n305 = call <vilib>:"Beep.vi"() -> ()  [unwired: 3 in, 9 out]
                      n306 = Number To Decimal String(number=w531, width (-)=i16 1) -> (decimal integer string=w529:string)
                      n307 = Concatenate Strings("Formed tether in ", w529, " attempt(s)." ("string")) -> (w526:string)
                      n308 = local read "Messages"() -> (w533:string)
                      n309 = local write "Fish for Tether"(w535) -> ()
                      n310 = call "Update messages.vi"("Message to add"=w526, "Old message string"=w533) -> ("New message string"=w532:string)
                      n311 = local write "Messages"(w532) -> ()
                      n312 = Get Date/Time In Seconds() -> (seconds since 1Jan1904=→"Time tether formed":timestamp)
                      n313 = local read "Flow ON during cal?"() -> (w523:bool)
                      n314 = property on="Sample Channel\nFlow" class="Bool (strict)"("Val(Sgnl)"=w523) -> (error out=w524:errorcluster)  [unwired: 2 in, 1 out]
                      n315 = case shown="\"2\", \"3\", \"4\", \"5\", \"6\"" "Then..." {
                        selector: "Then..." -> [_ w539]
                        tunnel: w536 -> [w538 _]
                        tunnel: w524 -> [_ _]
                        frame "1", Default {
                          n316 = property on="BD 1 Frequency 1 (MHz)" class="DigNum (strict)"("Val(Sgnl)"=w538) -> ()  [unwired: 2 in, 2 out]
                        }
                        frame "2", "3", "4", "5", "6" {
                          n317 = flat-sequence {
                            tunnel: w539 -> [w541]
                            frame #0 {
                              n318 = property on="Trap Delta (MHz)" class="DigNum (strict)"("Val(Sgnl)"="Move to Delta 1 (MHz)") -> ()  [unwired: 2 in, 2 out]
                            }
                            frame #1 {
                              n319 = case shown="\"5\", \"6\"" w541 {
                                selector: w541 -> [w544 w554 _]
                                frame "3", "4" {
                                n320 = flat-sequence {
                                tunnel: w544 -> [w545]
                                tunnel: [w545] -> w542
                                tunnel: [w547] -> w543
                                tunnel: w542 -> [w547]
                                tunnel: w543 -> [w551]
                                frame #0 {
                                n321 = property on="Green Laser ON/Interlacing" class="Bool (strict)"("Val(Sgnl)"=TRUE ("Value (Signaling)")) -> ()  [unwired: 2 in, 2 out]
                                }
                                frame #1 {
                                n322 = Multiply(x="Wait Before Save (s)", y=u32 1000 ("x")) -> (x*y=w549:u32)
                                n323 = Wait (ms)(milliseconds to wait=w549) -> ()  [unwired: 1 out]
                                }
                                frame #2 {
                                n324 = property on="Start Saving" class="Bool (strict)"("Value"=TRUE ("Start Saving")) -> ()  [unwired: 2 in, 2 out]
                                n325 = case shown="\"4\"" w551 {
                                frame Default {
                                }
                                frame "4" {
                                n326 = property on="Fl. Triggered..." class="Bool (strict)"("Val(Sgnl)"=TRUE ("Value (Signaling)")) -> ()  [unwired: 2 in, 2 out]
                                }
                                }
                                }
                                }
                                }
                                frame "5", "6" {
                                n327 = stacked-sequence {
                                tunnel: w554 -> [_ _ _ _ _ _ w566]
                                frame #0 {
                                n328 = Replace Array Subset(array=u32[] [0] ("Index Values"), new element="Raster Set Upon Tether", index=0) -> (w555:u32[])
                                n329 = property on="Saved AOD Raster Scan Parameter Sets" class="Arr (strict)"("Index Values"=w555) -> ()  [unwired: 2 in, 2 out]
                                }
                                frame #1 {
                                n330 = Wait (ms)(milliseconds to wait=u32 500) -> ()  [unwired: 1 out]
                                }
                                frame #2 {
                                n331 = property on="Load parameters" class="Bool (strict)"("Val(Sgnl)"=TRUE ("Value (Signaling)")) -> ()  [unwired: 2 in, 2 out]
                                n332 = case shown="True" "Green ON During Raster" {
                                frame False {
                                }
                                frame True {
                                n333 = property on="Green Laser ON/Interlacing" class="Bool (strict)"("Val(Sgnl)"=TRUE ("Value (Signaling)")) -> ()  [unwired: 2 in, 2 out]
                                }
                                }
                                }
                                frame #3 {
                                n334 = Wait (ms)(milliseconds to wait=u32 500) -> ()  [unwired: 1 out]
                                }
                                frame #4 {
                                n335 = property on="Trap Raster Scan" class="Bool (strict)"("Val(Sgnl)"=TRUE ("Value (Signaling)")) -> ()  [unwired: 2 in, 2 out]
                                }
                                frame #5 {
                                n336 = Wait (ms)(milliseconds to wait=u32 2000) -> ()  [unwired: 1 out]
                                }
                                frame #6 {
                                n337 = flat-sequence {
                                tunnel: w566 -> [w573]
                                frame #0 {
                                n338 = while {
                                stop <- w569 stop-if-true
                                n339 = local read "Raster Scanning..."() -> (w568:bool)
                                n340 = local read "Saving..."() -> (w571:bool)
                                n341 = Wait (ms)(milliseconds to wait=u32 100) -> ()  [unwired: 1 out]
                                n342 = Not(x=w571) -> (.not. x?=w570:bool)
                                n343 = Not(x=w568) -> (.not. x?=w567:bool)
                                n344 = And(x=w570, y=w567) -> (x .and. y?=w569:bool)
                                }
                                }
                                frame #1 {
                                n345 = local read "Tether"() -> (w574:bool)
                                n346 = case shown="True" w574 {
                                tunnel: w573 -> [_ w576]
                                frame False {
                                n347 = property on="Fish for Tether" class="Bool (strict)"("Val(Sgnl)"="Fish again after \nraster break?") -> ()  [unwired: 2 in, 2 out]
                                }
                                frame True {
                                n348 = stacked-sequence {
                                tunnel: w576 -> [_ w580 _ _]
                                frame #0 {
                                n349 = property on="Trap Delta (MHz)" class="DigNum (strict)"("Val(Sgnl)"="Move to Delta 2 (MHz)") -> ()  [unwired: 2 in, 2 out]
                                n350 = case shown="True" "Flow ON after\ntether testing?" {
                                frame False {
                                }
                                frame True {
                                n351 = property on="Sample Channel\nFlow" class="Bool (strict)"("Val(Sgnl)"=TRUE ("Value (Signaling)")) -> ()  [unwired: 2 in, 2 out]
                                }
                                }
                                }
                                frame #1 {
                                n352 = flat-sequence {
                                tunnel: w580 -> [w582]
                                frame #0 {
                                n353 = Wait (ms)(milliseconds to wait=u32 500) -> ()  [unwired: 1 out]
                                }
                                frame #1 {
                                n354 = case shown="\"6\"" w582 {
                                frame Default {
                                }
                                frame "6" {
                                n355 = property on="Green Laser ON/Interlacing" class="Bool (strict)"("Val(Sgnl)"=TRUE ("Green Laser ON/Interlacing")) -> ()  [unwired: 2 in, 2 out]
                                }
                                }
                                }
                                frame #2 {
                                n356 = Wait (ms)(milliseconds to wait=u32 500) -> ()  [unwired: 1 out]
                                }
                                frame #3 {
                                n357 = local write "Start Saving"("Save at end (5, 6)") -> ()
                                }
                                }
                                }
                                frame #2 {
                                n358 = local read "Bead Sep. Int. Time (s)"() -> (w588:dbl)
                                n359 = Multiply(x=w588, y=1000.0) -> (x*y=w587:dbl)
                                n360 = Wait (ms)(milliseconds to wait=w587) -> ()  [unwired: 1 out]
                                }
                                frame #3 {
                                n361 = property on="Remove Offset" class="Bool (strict)"("Val(Sgnl)"=TRUE ("Value (Signaling)")) -> ()  [unwired: 2 in, 2 out]
                                }
                                }
                                }
                                }
                                }
                                }
                                }
                                }
                                }
                                frame "2", Default {
                                }
                              }
                            }
                          }
                        }
                      }
                      "Tether" <- "Tether Alarm?"
                    }
                  }
                }
                frame #2 {
                  n362 = local read "Oscillate Set 1"() -> (w595:bool)
                  n363 = local read "Stop All"() -> (w593:bool)
                  n364 = Or(x=w595, y=w590) -> (x .or. y?=w592:bool)
